vi "Read Medio Comunicacion.vi"(8 "error in (no error)":errorcluster, 11 "Instrumento in":refnum<class "Instrumento.lvclass">) -> (0 "error out":errorcluster, 2 "Medio Comunicacion":string, 3 "Instrumento out":refnum<class "Instrumento.lvclass">)   [LabVIEW 2020, in "Instrumento.lvclass"]
uses:
  Instrumento.lvclass
  Instrumento.lvclass/Instrumento.ctl
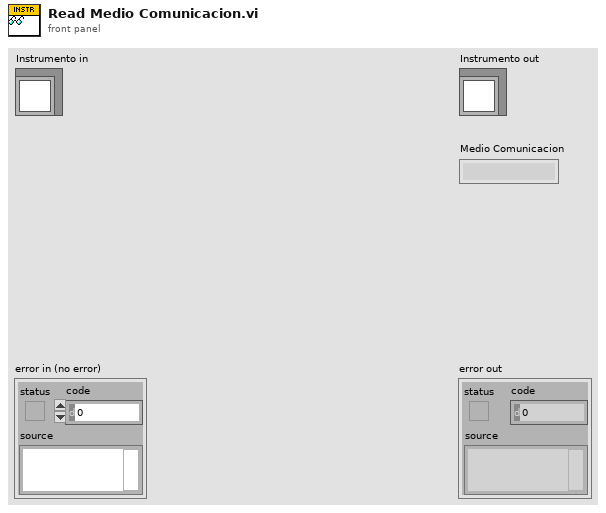
[diagram p1: front panel]
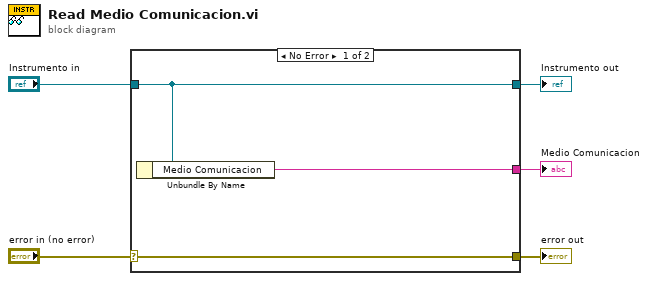
[diagram p0: block diagram]
diagram:
  n1 = case shown="No Error" "error in (no error)" {
    selector: "error in (no error)" -> [w8 w9]
    tunnel: [w8 w9] -> w4
    tunnel: [w7 w10] -> w2
    tunnel: "Instrumento in" -> [w7 w10]
    tunnel: [w6 _] -> w1
    frame No Error {
      n2 = Unbundle By Name(w7) -> ("Medio Comunicacion"=w6:string)
    }
    frame Error {
    }
  }
  "error out" <- w4
  "Instrumento out" <- w2
  "Medio Comunicacion" <- w1
